vi "Write Trigger Config In.vi"(8 "error in (no error)":errorcluster, 10 "Trigger Config In":variant, 11 "DIO in":refnum<class "DIO.lvclass">) -> (0 "error out":errorcluster, 3 "DIO out":refnum<class "DIO.lvclass">)   [LabVIEW 2015, in "DIO.lvclass"]
uses:
  DIO.lvclass
  DIO.lvclass/DIO.ctl
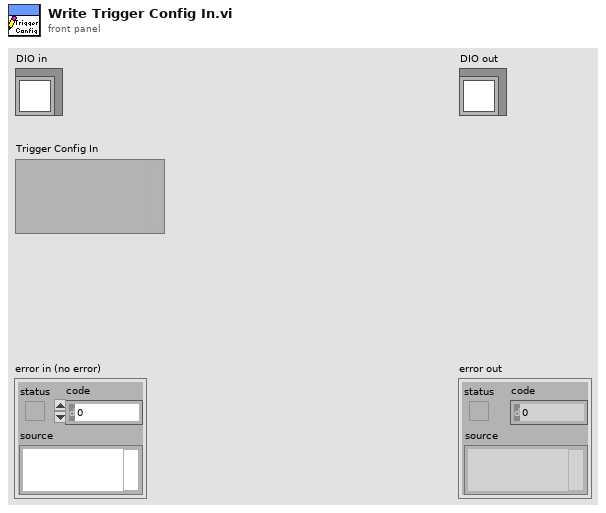
[diagram p1: front panel]
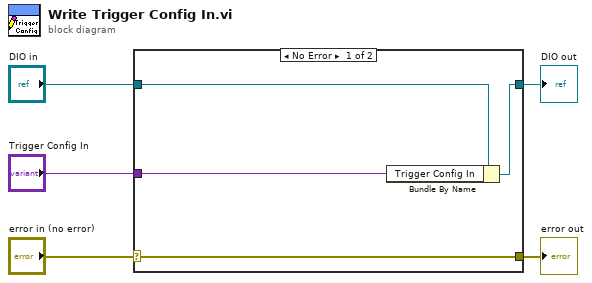
[diagram p0: block diagram]
diagram:
  n1 = case shown="No Error" "error in (no error)" {
    selector: "error in (no error)" -> [w9 w10]
    tunnel: [w9 w10] -> w4
    tunnel: [w7 w11] -> w2
    tunnel: "DIO in" -> [w8 w11]
    tunnel: "Trigger Config In" -> [w6 _]
    frame No Error {
      n2 = Bundle By Name(cluster=w8, "Trigger Config In"=w6) -> (w7:refnum<class "DIO.lvclass">)
    }
    frame Error {
    }
  }
  "error out" <- w4
  "DIO out" <- w2
